vi "Do.vi"(8 "error in (no error)":errorcluster, 10 "Actor in":refnum<class "Actor.lvclass">, 11 "Set Output Lines Msg":refnum<class "Set Output Lines Msg.lvclass">) -> (0 "error out":errorcluster, 2 "Actor out":refnum<class "Actor.lvclass">)   [LabVIEW 2016, in "BNT_DAQmx.lvlib" / "Set Output Lines Msg.lvclass"]
doc: "This VI delivers the message to the actor by calling the appropriate method(s) on the actor."
uses:
  Set Output Lines Msg.lvclass
  <vilib>/ActorFramework/Actor/Actor.lvclass
  C:/User/Brand/LVP/BNT/EQCR/Packages/CSPP_Core/Actors/CS++PVMonitor Messages/CS++PVUpdate Msg/CS++PVUpdate Msg.lvclass
  BNT_DAQmx-MCSV/BNT_DAQmx-MCSV.lvclass
  C:/Program Files (x86)/National Instruments/LabVIEW 2016/vi.lib/ActorFramework/Actor/Actor.lvclass
  CSPP_Core/Actors/CS++PVMonitor Messages/CS++PVUpdate Msg/CS++PVUpdate Msg.lvclass/CS++PVUpdate Msg.ctl
  CSPP_Core/Classes/CS++ProcessVariables/ProcessVariable/PV.lvclass/PV.ctl
  Set Output Lines Msg.lvclass/Set Output Lines Msg.ctl
  CSPP_Core/Classes/CS++ProcessVariables/ProcessVariable/PV.lvclass
  CSPP_Core/Actors/CS++PVMonitor Messages/CS++PVUpdate Msg/CS++PVUpdate Msg.lvclass
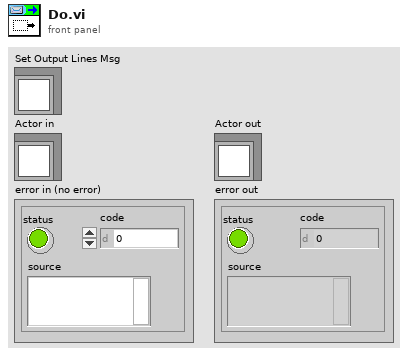
[diagram p1: front panel]
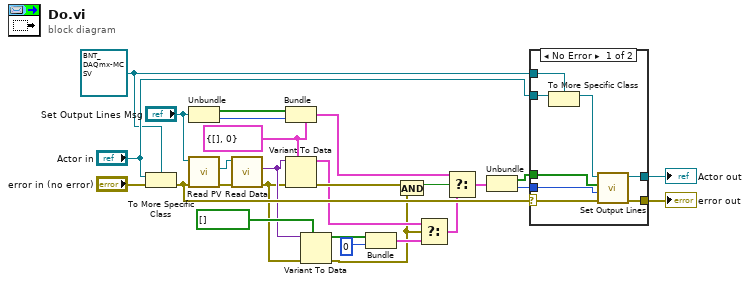
[diagram p0: block diagram]
diagram:
  w19 = cluster{"DO Lines":bool[], "Start Index":i32} {"DO Lines"=[], "Start Index"=0} ("Type")
  w23 = refnum<class "BNT_DAQmx-MCSV.lvclass"> refnum ("Actor in")
  n1 = To More Specific Class(target class=w23, reference="Actor in", error in="error in (no error)") -> (error out=w15:errorcluster)  [unwired: 1 out]
  n2 = Unbundle ("Pre-Unbundler")("Set Output Lines Msg") -> (w12:bool[], w11:i32)
  n3 = call "Read PV.vi"("error in (no error)"=w15, "CS++PVUpdate Msg in"="Set Output Lines Msg") -> ("error out"=w22:errorcluster, "PV"=w18:refnum<class "PV.lvclass">)  [unwired: 7 in, 1 out]
  n4 = call "Read Data.vi"("error in (no error)"=w22, "PV in"=w18) -> ("error out"=w5:errorcluster, "Data"=w6:variant)  [unwired: 7 in, 1 out]
  n5 = Bundle ("Pre-Bundler")(cluster=w19, "DO Lines"=w12, "Start Index"=w11) -> (w20:cluster{"DO Lines":bool[], "Start Index":i32})
  n6 = Variant To Data(error in=w5, type=w19, Variant=w6) -> (data=w4:cluster{"DO Lines":bool[], "Start Index":i32}, error out=w21:errorcluster)
  n7 = Variant To Data(error in=w5, type=bool[] [] ("Values"), Variant=w6) -> (data=w8:bool[], error out=w1:errorcluster)
  n8 = Bundle ("Pre-Bundler")("Values"=w8, "Start Index"=0) -> (w10:cluster{"Values":bool[], "Start Index":i32})  [unwired: 1 in]
  n9 = And(x=w21, y=w1) -> (x .and. y?=w2:bool)
  n10 = Select ("MainSelect")(t=w4, s=w1, f=w10) -> (s? t:f=w3:cluster{"Values":bool[], "Start Index":i32})
  n11 = Select ("MainSelect")(t=w20, s=w2, f=w3) -> (s? t:f=w17:cluster{"Values":bool[], "Start Index":i32})
  n12 = Unbundle ("Main-Unbundler")(w17) -> ("Values"=w14:bool[], "Start Index"=w13:i32)
  n13 = case shown="No Error" w15 {
    selector: w15 -> [w33 w37]
    tunnel: [w35 w37] -> w26
    tunnel: [w34 w36] -> w25
    tunnel: "Actor in" -> [w32 w36]
    tunnel: w23 -> [w31 _]
    tunnel: w14 -> [w29 _]
    tunnel: w13 -> [w28 _]
    frame No Error {
      n14 = To More Specific Class(target class=w31, reference=w32) -> (specific class reference=w30:refnum<class "BNT_DAQmx-MCSV.lvclass">)  [unwired: 1 in, 1 out]
      n15 = call "Set Output Lines.vi"("Error In"=w33, "Start Index"=w28, "DO Lines"=w29, "BNT_DAQmx-MCSV in"=w30) -> ("Error Out"=w35:errorcluster, "BNT_DAQmx-MCSV out"=w34:refnum<class "BNT_DAQmx-MCSV.lvclass">)  [unwired: 6 in]
    }
    frame Error {
    }
  }
  "error out" <- w26
  "Actor out" <- w25
